vi "Sinusoidal.vi"() -> ()   [LabVIEW 2015]
panel:
  out "Numeric":i32
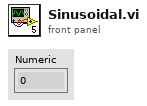
[diagram p1: front panel]
types:
  T1 = enum16{"Full", "Half", "Quarter", "Eighth", "Sixteenth"}
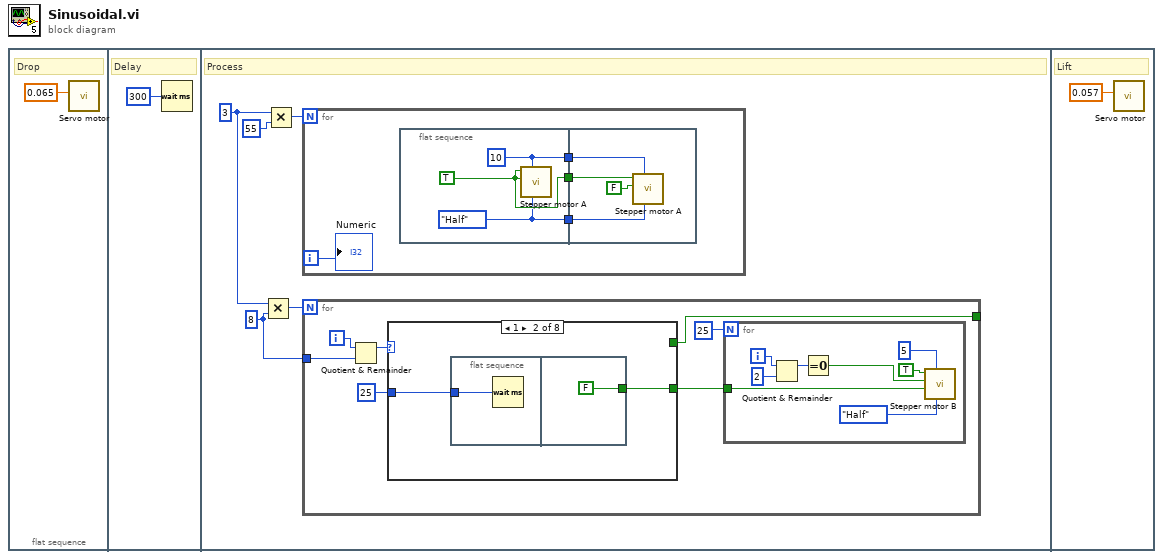
[diagram p0: block diagram]
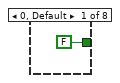
[diagram p2: hidden frame]
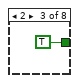
[diagram p3: hidden frame]
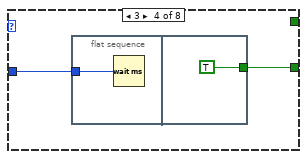
[diagram p4: hidden frame]
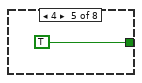
[diagram p5: hidden frame]
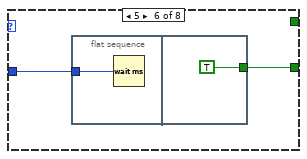
[diagram p6: hidden frame]
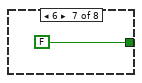
[diagram p7: hidden frame]
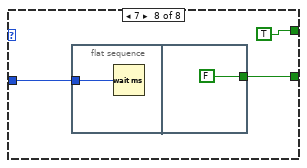
[diagram p8: hidden frame]
diagram:
  n1 = flat-sequence {
    frame #0 {
      # "Drop"
      n2 = call "Servo motor.vi"("Duty Cycle"=0.065) -> ()  [unwired: 9 in, 2 out]
    }
    frame #1 {
      # "Delay"
      n3 = Wait (ms)(milliseconds to wait=u32 300) -> ()  [unwired: 1 out]
    }
    frame #2 {
      w3 = 8 ("y")
      w4 = 3
      # "Process"
      n4 = Multiply(x=w4, y=w3) -> (x*y=w7:i32)
      n5 = Multiply(x=w4, y=55 ("Numeric")) -> (x*y=w6:i32)
      n6 = for {
        N: w6 -> [_]
        i -> [w44]
        n7 = flat-sequence {
          tunnel: [w50] -> w47
          tunnel: [w49] -> w46
          tunnel: [w48] -> w45
          tunnel: w47 -> [w54]
          tunnel: w46 -> [w52]
          tunnel: w45 -> [w51]
          frame #0 {
            w48 = T1."Half" ("Microstep size")
            w49 = u32 10 ("Speed")
            w50 = TRUE ("Enable (C/DIO2 (DIO2))")
            n8 = call "Stepper motor A.vi"("Microstep size"=w48, "Speed"=w49, "Step (C/DIO3 (DIO3))"=w50, "Enable (C/DIO2 (DIO2))"=w50) -> ()  [unwired: 7 in, 1 out]
          }
          frame #1 {
            n9 = call "Stepper motor A.vi"("Microstep size"=w51, "Speed"=w52, "Step (C/DIO3 (DIO3))"=FALSE, "Enable (C/DIO2 (DIO2))"=w54) -> ()  [unwired: 7 in, 1 out]
          }
        }
        "Numeric" <- w44
      }
      n10 = for {
        N: w7 -> [_]
        tunnel: w3 -> [w9]
        tunnel: [w8] -> _
        i -> [w11]
        n11 = Quotient & Remainder(x=w11, y=w9) -> (x-y*floor(x/y)=w10:i32)  [unwired: 1 out]
        n12 = case shown="1" w10 {
          tunnel: [FALSE w17 TRUE w22 TRUE w27 FALSE w33] -> w13
          tunnel: u32 25 -> [_ w16 _ w21 _ w26 _ w32]
          tunnel: [_ _ _ _ _ _ _ TRUE] -> w8
          frame 0, Default {
          }
          frame 1 {
            n13 = flat-sequence {
              tunnel: w16 -> [w18]
              tunnel: [FALSE] -> w17
              frame #0 {
                n14 = Wait (ms)(milliseconds to wait=w18) -> ()  [unwired: 1 out]
              }
              frame #1 {
              }
            }
          }
          frame 2 {
          }
          frame 3 {
            n15 = flat-sequence {
              tunnel: w21 -> [w23]
              tunnel: [TRUE] -> w22
              frame #0 {
                n16 = Wait (ms)(milliseconds to wait=w23) -> ()  [unwired: 1 out]
              }
              frame #1 {
              }
            }
          }
          frame 4 {
          }
          frame 5 {
            n17 = flat-sequence {
              tunnel: w26 -> [w28]
              tunnel: [TRUE] -> w27
              frame #0 {
                n18 = Wait (ms)(milliseconds to wait=w28) -> ()  [unwired: 1 out]
              }
              frame #1 {
              }
            }
          }
          frame 6 {
          }
          frame 7 {
            n19 = flat-sequence {
              tunnel: w32 -> [w34]
              tunnel: [FALSE] -> w33
              frame #0 {
                n20 = Wait (ms)(milliseconds to wait=w34) -> ()  [unwired: 1 out]
              }
              frame #1 {
              }
            }
          }
        }
        n21 = for {
          N: 25 -> [_]
          tunnel: w13 -> [w38]
          i -> [w39]
          n22 = Quotient & Remainder(x=w39, y=2) -> (x-y*floor(x/y)=w41:i32)  [unwired: 1 out]
          n23 = Equal To 0?(x=w41) -> (x = 0?=w40:bool)
          n24 = call "Stepper motor B.vi"("Microstep size"=T1."Half", "Speed"=u32 5, "Direction (A/DIO5 (Pin 21))"=w38, "Step (A/DIO4 (Pin 19))"=w40, "Enable (A/DIO0 (Pin 11))"=TRUE ("Enable (C/DIO2 (DIO2))")) -> ()  [unwired: 5 in, 2 out]
        }
      }
    }
    frame #3 {
      # "Lift"
      n25 = call "Servo motor.vi"("Duty Cycle"=0.057) -> ()  [unwired: 9 in, 2 out]
    }
  }
